vi "Returning A Value 2D Array Of Integers.vi"(10 "cols":i32, 11 "rows":i32) -> (3 "function return":cluster{})   [LabVIEW 2018, in "ParsingDataSampleDLL.lvlib"]
doc: "__declspec(dllexport) int** ReturningAValue_2DArrayOfIntegers (int rows, int cols);"
uses:
  ParsingDataSampleDLL.lvlib
  ni_reference_vs/Debug/ParsingDataSampleDLL.dll
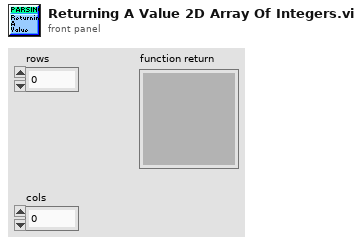
[diagram p1: front panel]
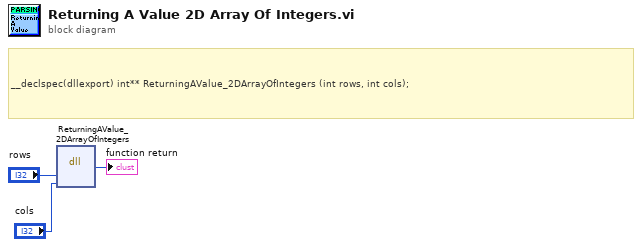
[diagram p0: block diagram]
diagram:
  # "__declspec(dllexport) int** ReturningAValue_2DArrayOfIntegers (int rows, int cols);"
  n1 = dll-call lib="C:/Users/celit/Documents/GitHub/Labview_Python_DLL_Call/ni_reference_vs/Debug/ParsingDataSampleDLL.*" fn="ReturningAValue_2DArrayOfIntegers"("rows"="rows", "cols"="cols") -> (→"function return":u32)  [unwired: 5 in, 2 out]
